vi "Read Serial Data Unit.vi"(8 "error in (no error)":errorcluster, 11 "Serial Master in":refnum<class "Serial Master.lvclass">) -> (0 "error out":errorcluster, 2 "Serial Data Unit":refnum<class "Serial Data Unit.lvclass">, 3 "Serial Master out":refnum<class "Serial Master.lvclass">)   [LabVIEW 2012, in "Serial Master.lvclass"]
uses:
  Serial Master.lvclass
  Transmission Data Unit/Serial Interface/Serial Data Unit.lvclass
  Serial Master.lvclass/Serial Master.ctl
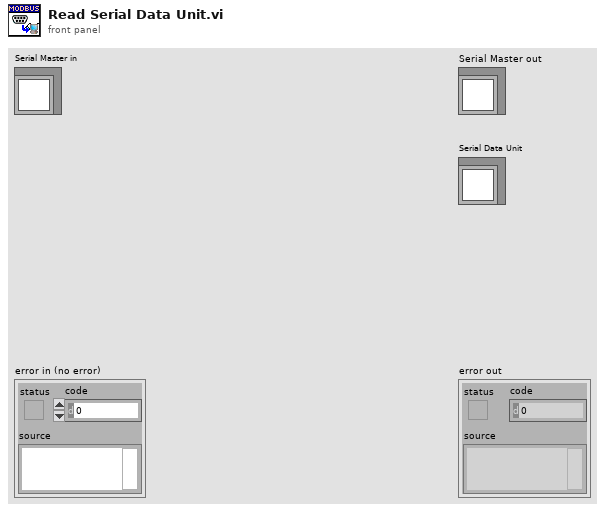
[diagram p1: front panel]
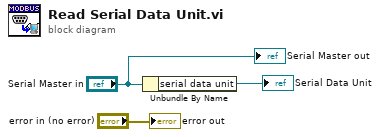
[diagram p0: block diagram]
diagram:
  n1 = Unbundle By Name("Serial Master in") -> ("serial data unit"=→"Serial Data Unit":refnum<class "Serial Data Unit.lvclass">)
  "error out" <- "error in (no error)"
  "Serial Master out" <- "Serial Master in"
